vi "MGI Log Error Occurrence[].vi"(8 "error in (no error)":errorcluster, 10 "Error Occurence[]":errorcluster[](array[cluster]), 11 "MGI Error Reporter Base in":refnum<class "MGI Error Reporter Base.lvclass">) -> (0 "error out":errorcluster, 3 "MGI Error Reporter Base out":refnum<class "MGI Error Reporter Base.lvclass">)   [LabVIEW 2020, in "MGI Error Reporter Base.lvclass"]
doc: "Write the error occurrence array to a file within the specified directory. Files are named using creation date of the form:\nYYYY-mm-dd HHMMSS Errors.txt\nChild classes may override this VI and perform their own file I/O. \n\nAuthored by Shawn Walpole\nsupport@mooregoodideas.com\nwww.mooregoodideas.com\n\nCopyright (c) 2013, Moore Good Ideas, Inc.\n\nAll rights reserved.\n\nRedistribution and use in source and binary forms, with or without modification, are permitted provided that the following conditions are met:\n\n * Redistributions of source code must retain the above copyright notice, this list of conditions and the following disclaimer.\n * Redistributions in binary form must reproduce the above copyright notice, this list of conditions and the following disclaimer in the documentation and/or other materials provided with the distribution.\n * Neither the name of Moore Good Ideas, Inc. nor the names of its contributors may be used to endorse or promote products derived from this software without specific prior written permission.\n\nTHIS SOFTWARE IS PROVIDED BY THE COPYRIGHT HOLDERS AND CONTRIBUTORS \"AS IS\" AND ANY EXPRESS OR IMPLIED WARRANTIES, INCLUDING, BUT NOT LIMITED TO, THE IMPLIED WARRANTIES OF MERCHANTABILITY AND FITNESS FOR A PARTICULAR PURPOSE ARE DISCLAIMED. IN NO EVENT SHALL THE COPYRIGHT OWNER OR CONTRIBUTORS BE LIABLE FOR ANY DIRECT, INDIRECT, INCIDENTAL, SPECIAL, EXEMPLARY, OR CONSEQUENTIAL DAMAGES (INCLUDING, BUT NOT LIMITED TO, PROCUREMENT OF SUBSTITUTE GOODS OR SERVICES; LOSS OF USE, DATA, OR PROFITS; OR BUSINESS INTERRUPTION) HOWEVER CAUSED AND ON ANY THEORY OF LIABILITY, WHETHER IN CONTRACT, STRICT LIABILITY, OR TORT (INCLUDING NEGLIGENCE OR OTHERWISE) ARISING IN ANY WAY OUT OF THE USE OF THIS SOFTWARE, EVEN IF ADVISED OF THE POSSIBILITY OF SUCH DAMAGE."
uses:
  <userlib>/_MGI/Error Reporter/MGI Error Reporter Base/MGI Error Reporter Base.lvclass
  <userlib>/_MGI/Error Reporter/MGI Error Reporter Base/MGI Error Reporter Base.lvclass/MGI Error Reporter Base.ctl
  <userlib>/_MGI/File/MGI Create Directory Chain Behavior Enum.ctl
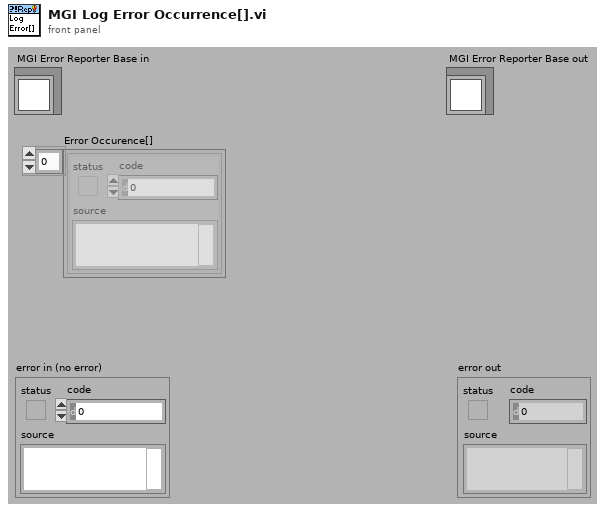
[diagram p1: front panel]
types:
  T1 = typedef "MGI Create Directory Chain Behavior Enum.ctl" = enum16{"Auto Detect", "Path Contains a File", "Path Does Not Contain a File"}
  T2 = enum16{"open", "replace", "create", "open or create", "replace or create", "replace or create with confirmation"}
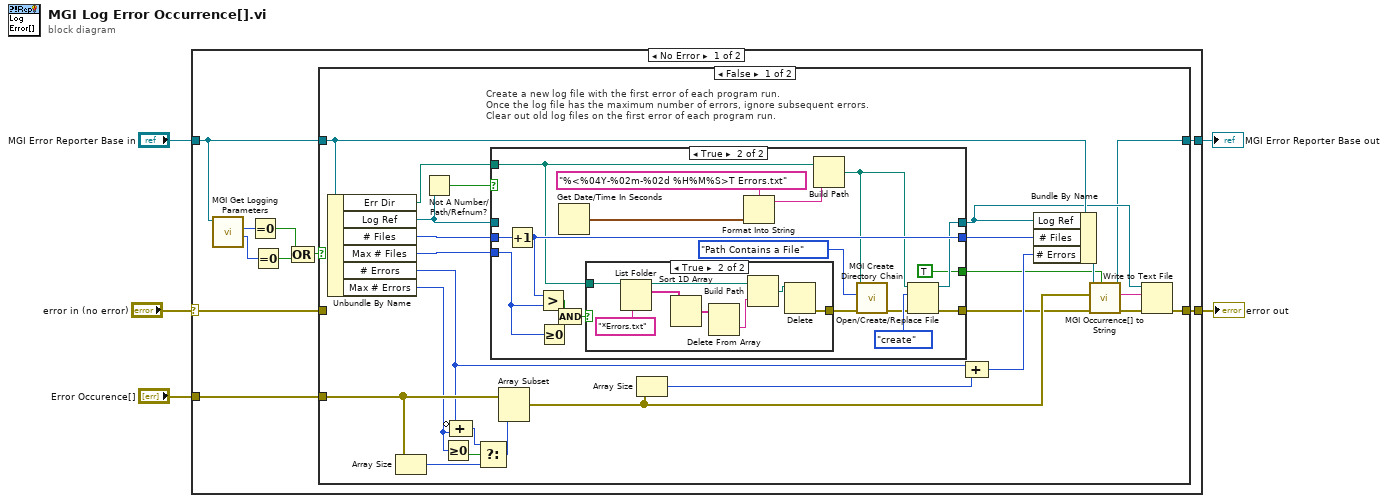
[diagram p0: block diagram]
diagram:
  n1 = case shown="No Error" "error in (no error)" {
    selector: "error in (no error)" -> [w12 w72]
    tunnel: "MGI Error Reporter Base in" -> [w8 w71]
    tunnel: [w15 w72] -> w4
    tunnel: "Error Occurence[]" -> [w14 _]
    tunnel: [w13 w71] -> w2
    frame No Error {
      n2 = call <userlib>:"MGI Get Logging Parameters.vi"("MGI Error Reporter Base"=w8) -> ("Max # Log Files"=w7:i32, "Max # Errors to Log"=w6:i32)  [unwired: 9 out]
      n3 = Equal To 0?(x=w6) -> (x = 0?=w10:bool)
      n4 = Equal To 0?(x=w7) -> (x = 0?=w11:bool)
      n5 = Compound Arithmetic op=OR(w10, w11) -> (w9:bool)
      n6 = case shown="False" w9 {
        tunnel: w8 -> [w40 w70]
        tunnel: [w31 w69] -> w15
        tunnel: w14 -> [w30 _]
        tunnel: [w23 w70] -> w13
        tunnel: w12 -> [_ w69]
        frame False {
          # "Create a new log file with the first error of each program run.\nOnce the log file has the maximum number of errors, ignore subsequent errors.\nClear out old log files on the first error of each program run."
          n7 = Unbundle By Name(w40) -> ("Err Dir"=w19:path, "Log Ref"=w33:refnum<file>, "# Files"=w35:i32, "Max # Files"=w34:i32, "# Errors"=w18:i32, "Max # Errors"=w17:i32)
          n8 = Array Size(array=w30) -> (size(s)=w36:i32)
          n9 = Not A Number/Path/Refnum?(number/path/refnum=w33) -> (NaN/Path/Refnum?=w16:bool)
          n10 = Greater Or Equal To 0?(x=w17) -> (x >= 0?=w38:bool)
          n11 = Compound Arithmetic op=ADD(invert w18, w17) -> (w37:i32)
          n12 = Select(t=w37, s=w38, f=w36) -> (s? t:f=w29:i32)
          n13 = case shown="True" w16 {
            tunnel: w35 -> [w41 w60]
            tunnel: w34 -> [_ w52]
            tunnel: w33 -> [w42 _]
            tunnel: [w42 w58] -> w28
            tunnel: [w41 w59] -> w32
            tunnel: [_ w57] -> w24
            tunnel: w19 -> [_ w49]
            tunnel: [_ TRUE] -> w20
            frame False {
            }
            frame True {
              n14 = Increment(x=w60) -> (x+1=w59:i32)
              n15 = Greater?(x=w59, y=w52) -> (0:w51:bool)
              n16 = Greater Or Equal To 0?(x=w52) -> (x >= 0?=w50:bool)
              n17 = Get Date/Time In Seconds() -> (seconds since 1Jan1904=w54:timestamp)
              n18 = Compound Arithmetic op=AND(w51, w50) -> (w48:bool)
              n19 = case shown="True" w48 {
                tunnel: w49 -> [_ w68]
                tunnel: [_ w64] -> w45
                frame False {
                }
                frame True {
                  n20 = List Folder(path=w68, pattern="*Errors.txt") -> (path out=w63:path, filenames=w66:string[])  [unwired: 1 in, 3 out]
                  n21 = Sort 1D Array(array=w66) -> (sorted array=w65:string[])
                  n22 = Delete From Array(array=w65) -> (deleted portion=w61:string)  [unwired: 2 in, 1 out]
                  n23 = Build Path(base path=w63, name or relative path=w61) -> (appended path=w62:path)
                  n24 = Delete(path (use dialog)=w62) -> (error out=w64:errorcluster)  [unwired: 1 in, 5 out]
                }
              }
              n25 = Format Into String(format string="%<%04Y-%02m-%02d %H%M%S>T Errors.txt", w54) -> (resulting string=w53:string)  [unwired: 2 in, 1 out]
              n26 = Build Path(base path=w49, name or relative path=w53) -> (appended path=w43:path)
              n27 = call <userlib>:"MGI Create Directory Chain.vi"("Error In"=w45, "File Presence (Auto Detect)"=MGI_Create_Directory_Chain_Behavior_Enum."Path Contains a File", "Path"=w43) -> ("Error Out"=w46:errorcluster)  [unwired: 8 out]
              n28 = Open/Create/Replace File(file path (use dialog)=w43, error in=w46, operation (0:open)=T2."create") -> (refnum out=w58:refnum<file>, error out=w57:errorcluster)  [unwired: 4 out]
            }
          }
          n29 = Array Subset(array=w30, length=w29) -> (w25:errorcluster[])  [unwired: 1 in]
          n30 = Array Size(array=w25) -> (size(s)=w27:i32)
          n31 = Compound Arithmetic op=ADD(w18, w27) -> (w39:i32)
          n32 = Bundle By Name(cluster=w40, "Log Ref"=w28, "# Files"=w32, "# Errors"=w39) -> (w26:refnum<class "MGI Error Reporter Base.lvclass">)
          n33 = call-dynamic "MGI Occurrence[] to String.vi"("Add Column Header? (F)"=w20, "error in (no error)"=w24, "Error[]"=w25, "MGI Error Reporter Base In"=w26) -> ("error out"=w21:errorcluster, "Delimited String"=w22:string, "MGI Error Reporter Base Out"=w23:refnum<class "MGI Error Reporter Base.lvclass">)  [unwired: 5 out]
          n34 = Write to Text File(file (use dialog)=w28, text=w22, error in=w21) -> (error out=w31:errorcluster)  [unwired: 3 out]
        }
        frame True {
        }
      }
    }
    frame Error {
    }
  }
  "error out" <- w4
  "MGI Error Reporter Base out" <- w2
